vi "Measurement Data Convert (Normal).vi"(8 "error in (no error)":errorcluster, 9 "Item Number Offset (1)":i32=1 min=1 max=255, 10 "Measurement Data (Empty)":string, 11 "VISA resource name":refnum<visa-resource-name>) -> (0 "error out":errorcluster, 1 "Measurement":dbl[](array[numeric]), 2 "Function":string[](array[string]), 3 "VISA resource name out":refnum<visa-resource-name>)   [LabVIEW 2021, in "Yokogawa WT1800 Series.lvlib"]
doc: "Transforms measurement datas into normal numeric values."
uses:
  <instrlib>/Yokogawa WT1800 Series/Yokogawa WT1800 Series.lvlib
  <instrlib>/Yokogawa WT1800 Series/Public/Action-Status/Query Numeric (Normal).vi
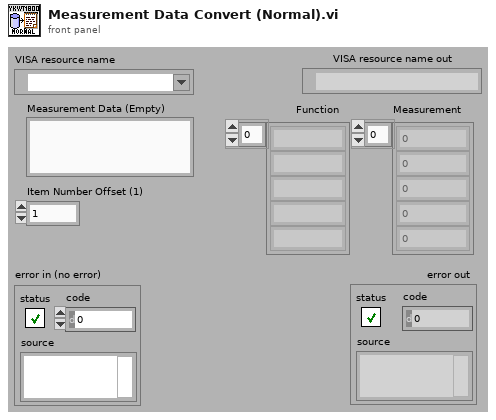
[diagram p1: front panel]
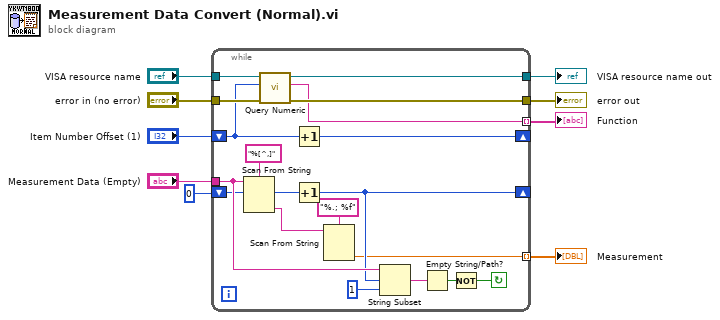
[diagram p0: block diagram]
diagram:
  n1 = while {
    tunnel: [w18] -> w3 mode=indexing
    tunnel: "Measurement Data (Empty)" -> [w23]
    shift-right: [w20] -> _
    shift-left: 0 -> [w22]
    tunnel: "VISA resource name" -> [w16]
    tunnel: "error in (no error)" -> [w15]
    shift-right: [w13] -> _
    shift-left: "Item Number Offset (1)" -> [w14]
    tunnel: [w12] -> w6
    tunnel: [w11] -> w5
    tunnel: [w10] -> w4 mode=indexing
    stop <- w25 continue-if-true
    n2 = Scan From String(format string="%[^,]", input string=w23, initial scan location=w22) -> (offset past scan=w21:u32, output 1=w19:string)  [unwired: 2 in, 2 out]
    n3 = call-poly <instrlib>:"Query Numeric.vi"("error in (no error)"=w15, "Item (1)"=w14, "VISA resource name"=w16) -> ("error out"=w11:errorcluster, "Function"=w10:string, "VISA resource name out"=w12:refnum<visa-resource-name>)  [unwired: 6 in]
    n4 = Increment(x=w14) -> (x+1=w13:i32)
    n5 = Increment(x=w21) -> (x+1=w20:u32)
    n6 = Scan From String(format string="%.; %f" ("形式文字列"), input string=w19) -> (output 1=w18:dbl)  [unwired: 3 in, 3 out]
    n7 = String Subset(string=w23, offset (0)=w20, length (rest)=1) -> (substring=w27:string)
    n8 = Empty String/Path?(string/path=w27) -> (empty?=w26:bool)
    n9 = Not(x=w26) -> (.not. x?=w25:bool)
  }
  "error out" <- w5
  "VISA resource name out" <- w6
  "Measurement" <- w3
  "Function" <- w4
